vi "Image.vi"(2 "XRef":refnum<vi>, 3 "State In":T1) -> (0 "Image":picture)   [LabVIEW 2012, in "CRefScripting.lvlib" / "CRef Label Node.xnode"]
doc: "This ability VI is used to describe your XNode's appearance. The origin of Image corresponds to the top-left corner of your XNode. The bounds of your XNode are used to crop this image. If you want LabVIEW to update your image, you need to inform it through the UpdateImage or UpdateImageAndBounds replies. Any areas where you do not draw are transparent, so regions intended to appear white should be explicitly drawn.\n \n Remember to localize any strings that are part of your image.\n\nDefault behavior: None.\n\nThis ability does not provide UI and OS messages are not handled."
uses:
  CRef Label Node.xnode
  State.ctl
  Core/Master Types.ctl
  <vilib>/picture/picture.llb/Draw True-Color Pixmap.vi
  CRef.lvlib
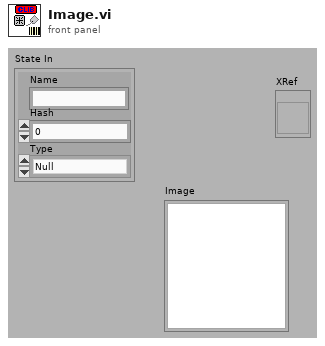
[diagram p1: front panel]
types:
  T1 = typedef "CRefScripting.lvlib/CRef Label Node.xnode/State.ctl" = cluster{"Name":string, "Hash":u32, "Type":T2}
  T2 = typedef "CRef.lvlib/Master Types.ctl" = enum8{"Null", "Boolean", "U8", "I8", "U16", "I16", "U32", "I32", "U64", "I64", "Single", "Double", "Extended", "CSG", "CDB", "CXT", "Boolean(Def)", "U8(Def)", "I8(Def)", "U16(Def)", "I16(Def)", "U32(Def)", "I32(Def)", "Reserved Def", "Reserved Def1", "Single(Def)", "Double(Def)", "Reserved Def2", "Reserved Def3", "Reserved Def4", "Reserved Def5", "Unsigned(Def)", "Signed(Def)", "Real(Def)", "Reserved Def6", "Numeric(Def)", "String"}
  T3 = typedef "imagedata.ctl" = cluster{"image type":i32, "image depth":i32, "image":u8[], "mask":u8[], "colors":u32[], "Rectangle":cluster{"left":i16, "top":i16, "right":i16, "bottom":i16}}
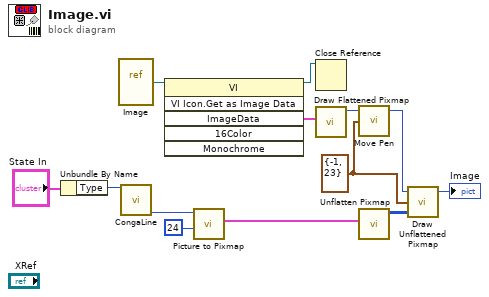
[diagram p0: block diagram]
diagram:
  w3 = cluster{"x":i16, "y":i16} {"x"=-1, "y"=23} ("Cluster")
  n1 = Unbundle By Name("State In") -> ("Type"=w11:T2)
  n2 = vi-ref "Image.vi"() -> (w13:refnum<vi>)
  n3 = call "CongaLine.vi"("Type"=w11) -> ("datatype image"=w4:picture)  [unwired: 11 in, 3 out]
  n4 = invoke class="VI" method="VI Icon.Get as Image Data"(reference=w13) -> (reference out=w10:refnum<vi>, "ImageData"=w2:T3)  [unwired: 5 in, 4 out]
  n5 = call <vilib>:"Picture to Pixmap.vi"("depth"=24, "picture"=w4) -> ("image data"=w6:T3)  [unwired: 8 in, 1 out]
  n6 = Close Reference(reference=w10) -> ()  [unwired: 1 in, 1 out]
  n7 = call <vilib>:"Draw Flattened Pixmap.vi"("image data"=w2) -> ("new picture"=w5:picture)  [unwired: 8 in]
  n8 = call <vilib>:"Move Pen.vi"("new position"=w3, "picture"=w5) -> ("new picture"=w9:picture)  [unwired: 3 in]
  n9 = call <vilib>:"Unflatten Pixmap.vi"("image data"=w6) -> ("24-bit pixmap"=w8:u32[][])  [unwired: 4 in, 6 out]
  n10 = call-poly <vilib>:"Draw Unflattened Pixmap.vi"("picture"=w9, "top left point(0, 0)"=w3, "data (RGB format)"=w8) -> ("new picture"=→"Image":picture)  [unwired: 6 in]
